vi "Change_Test_Mode.vi"() -> ()   [LabVIEW 2020]
panel:
  out "Which Button?":T1(ring)=enum."Center Button"
  in  "Test Mode":string
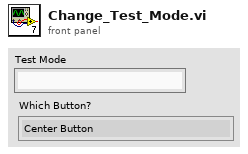
[diagram p1: front panel]
types:
  T1 = enum16{"Left Button", "Center Button", "Right Button", "Window Close"}
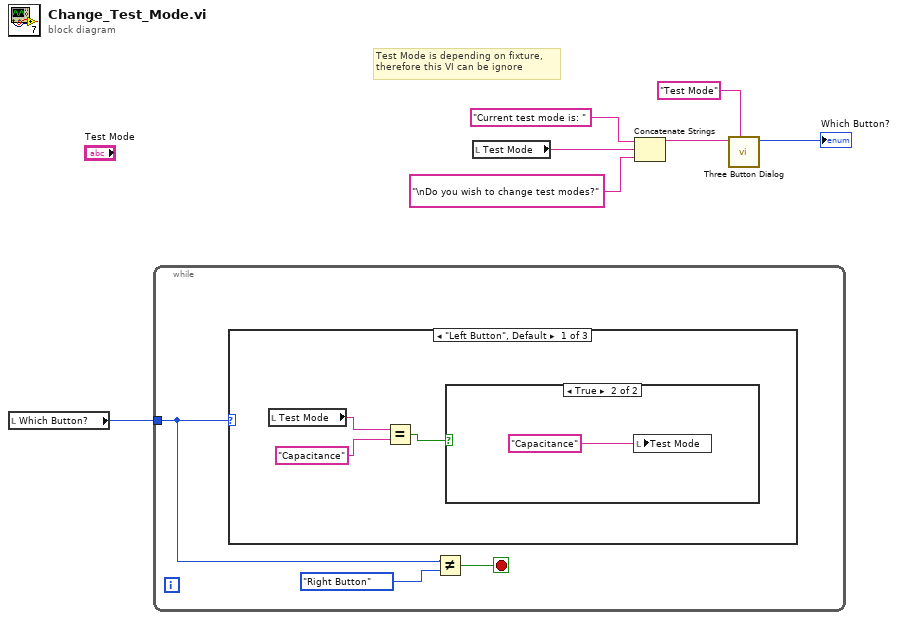
[diagram p0: block diagram]
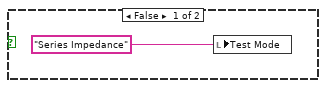
[diagram p2: hidden frame]
diagram:
  # "Test Mode is depending on fixture,\ntherefore this VI can be ignore"
  n1 = local read "Which Button?"() -> (w1:T1)
  n2 = while {
    tunnel: w1 -> [w10]
    stop <- w8 stop-if-true
    n3 = case shown="\"Left Button\", Default" w10 {
      frame "Left Button", Default {
        n4 = local read "Test Mode"() -> (w13:string)
        n5 = Equal?(x=w13, y="Capacitance") -> (x = y?=w11:bool)
        n6 = case shown="True" w11 {
          frame False {
            n7 = local write "Test Mode"("Series Impedance" ("Test Mode")) -> ()
          }
          frame True {
            n8 = local write "Test Mode"("Capacitance" ("Test Mode")) -> ()
          }
        }
      }
      frame "Right Button" {
      }
      frame "Center Button" {
      }
    }
    n9 = Not Equal?(x=w10, y=T1."Right Button") -> (x != y?=w8:bool)
  }
  n10 = local read "Test Mode"() -> (w6:string)
  n11 = Concatenate Strings("Current test mode is: " ("string"), w6, "\nDo you wish to change test modes?" ("string")) -> (w3:string)
  n12 = call <vilib>:"Three Button Dialog.vi"("Window Title (\"\")"="Test Mode" ("Window Title (\"\")"), "message"=w3) -> ("Which Button?"=→"Which Button?":T1)  [unwired: 9 in]
